vi "Read flows.vi"(8 "error in (no error)":errorcluster, 11 "Set Flows for Blue in":refnum<class "Set Flows for Blue.lvclass">) -> (0 "error out":errorcluster, 2 "flows":bool, 3 "Set Flows for Blue out":refnum<class "Set Flows for Blue.lvclass">)   [LabVIEW 2013, in "Set Flows for Blue.lvclass"]
uses:
  Set Flows for Blue.lvclass
  Set Flows for Blue.lvclass/Set Flows for Blue.ctl
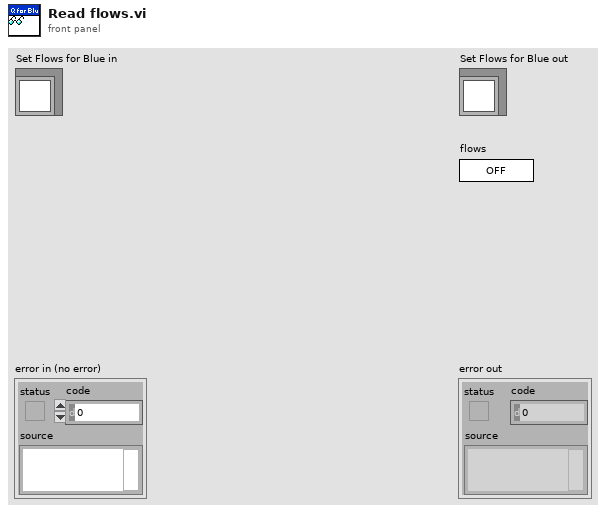
[diagram p1: front panel]
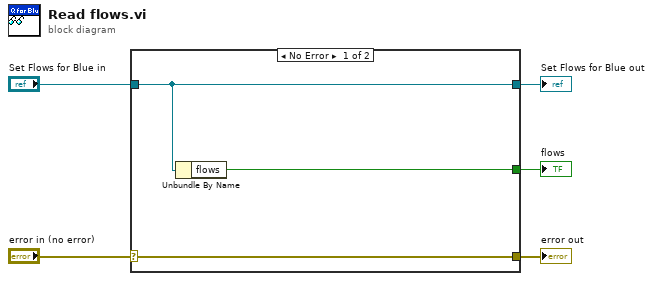
[diagram p0: block diagram]
diagram:
  n1 = case shown="No Error" "error in (no error)" {
    selector: "error in (no error)" -> [w8 w9]
    tunnel: [w8 w9] -> w4
    tunnel: [w7 w10] -> w2
    tunnel: "Set Flows for Blue in" -> [w7 w10]
    tunnel: [w6 _] -> w1
    frame No Error {
      n2 = Unbundle By Name(w7) -> ("flows"=w6:bool)
    }
    frame Error {
    }
  }
  "error out" <- w4
  "Set Flows for Blue out" <- w2
  "flows" <- w1
